vi "trigger_delay.vi"(3 "error in (no error)":errorcluster, 4 "Boolean":bool, 5 "VISA resource name":refnum<visa-resource-name>) -> (0 "error out":errorcluster, 2 "VISA resource name 2":refnum<visa-resource-name>)   [LabVIEW 2011]
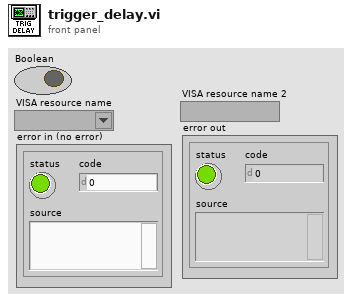
[diagram p1: front panel]
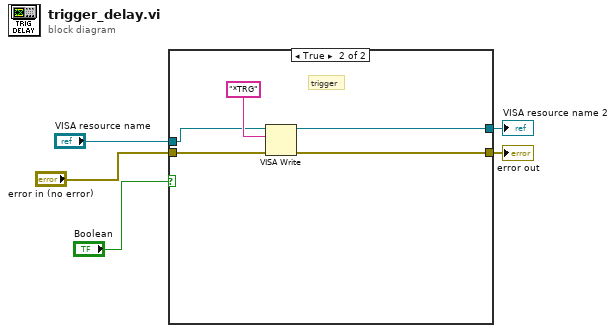
[diagram p0: block diagram]
diagram:
  n1 = case shown="True" "Boolean" {
    tunnel: "VISA resource name" -> [w7 w11]
    tunnel: "error in (no error)" -> [w6 w10]
    tunnel: [w7 w9] -> w2
    tunnel: [w6 w8] -> w1
    frame False {
      # "idle"
    }
    frame True {
      # "trigger"
      n2 = VISA Write(VISA resource name=w11, write buffer="*TRG" ("command"), error in (no error)=w10) -> (VISA resource name out=w9:refnum<visa-resource-name>, error out=w8:errorcluster)  [unwired: 1 out]
    }
  }
  "VISA resource name 2" <- w2
  "error out" <- w1
